vi "emi_Get system Info.vi"(11 "error in (no error)":errorcluster) -> (4 "Info retreived":bool, 8 "System Info":string, 15 "error out":errorcluster)   [LabVIEW 2011]
doc: "Reads a system infor summery from the OS.\n\nFor use in diagnostic files and such. \n\nThe system info generation takes a long time, so it should be run one time during startup. When it has run once, it will use the information retreived for all subsequent runs. First run: Long time. Secound run: No time.\nThe VI disregards the error input, and output. The asumption is that if this fails, the correct action is to do nothing. (The software should not exit due to this)."
uses:
  <vilib>/Utility/sysdir.llb/System Directory Type.ctl
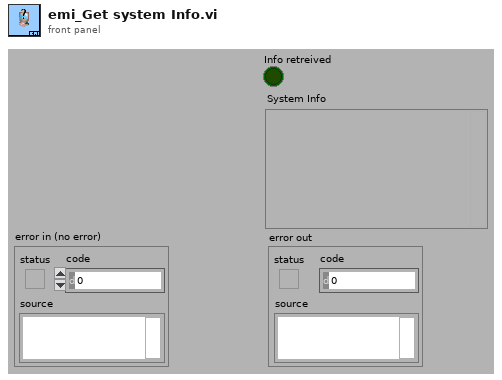
[diagram p1: front panel]
types:
  T1 = enum16{"open", "replace", "create", "open or create", "replace or create", "replace or create with confirmation"}
  T2 = typedef "System Directory Type.ctl" = i32
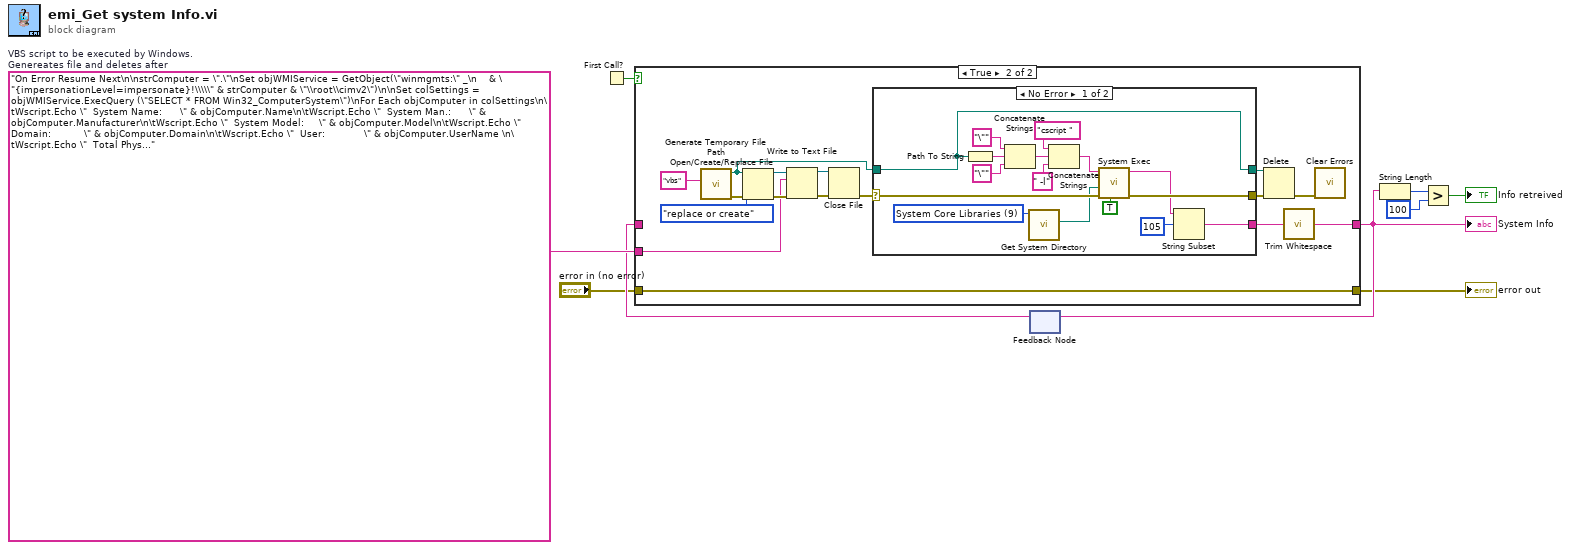
[diagram p0: block diagram]
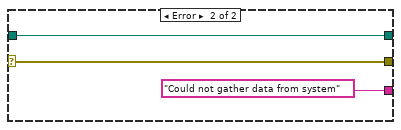
[diagram p3: hidden frame]
diagram:
  w9 = "On Error Resume Next\n\nstrComputer = \".\"\nSet objWMIService = GetObject(\"winmgmts:\" _\n    & \"{impersonationLevel=impersonate}!\\\\\" & strComputer & \"\\root\\cimv2\")\n\nSet colSettings = objWMIService.ExecQuery (\"SELECT * FROM Win32_ComputerSystem\")\nFor Each objComputer in colSettings\n\tWscript.Echo \"  System Name:      \" & objComputer.Name\n\tWscript.Echo \"  System Man.:      \" & objComputer.Manufacturer\n\tWscript.Echo \"  System Model:     \" & objComputer.Model\n\tWscript.Echo \"  Domain:           \" & objComputer.Domain\n\tWscript.Echo \"  User:             \" & objComputer.UserName \n\tWscript.Echo \"  Total Phys. Mem:  \" & objComputer.TotalPhysicalMemory\nNext\n\nSet colItems = objWMIService.ExecQuery(\"SELECT * FROM Win32_OperatingSystem\")\nFor Each objOperatingSystem in colItems \n \tWscript.Echo \"  Avail. Phys. Mem: \" & objOperatingSystem.FreePhysicalMemory\n \tWscript.Echo \"  Total Virt. Mem:  \" & objOperatingSystem.TotalVirtualMemorySize\n\tWscript.Echo \"  Avail. Virt. Mem: \" & objOperatingSystem.FreeVirtualMemory\n\tWscript.Echo \"  OS Name:          \" & objOperatingSystem.Name\n\tWscript.Echo \"  Version:          \" & objOperatingSystem.Version & \" SP: \" & objOperatingSystem.ServicePackMajorVersion & \".\" & objOperatingSystem.ServicePackMinorVersion\nNext\n\n\tWscript.Echo \" \"\n\nSet colItems = objWMIService.ExecQuery(\"Select * from Win32_SystemEnclosure\")\nFor Each objItem in colItems\n\tWscript.Echo \"  Part Numb.:       \" & objItem.PartNumber\n\tWscript.Echo \"  Serial Numb.:     \" & objItem.SerialNumber\n\tWscript.Echo \"  Asset tag.:       \" & objItem.SMBIOSAssetTag\nNext\n\n\tWscript.Echo \" \"\n\nSet colSettings = objWMIService.ExecQuery (\"SELECT * FROM Win32_ComputerSystem\")\nFor Each objComputer in colSettings\n\tWscript.Echo \"  Numb. CPU(s):     \" & objComputer.NumberOfProcessors\nNext\nSet colItems = objWMIService.ExecQuery(\"Select * from Win32_Processor\")\nFor Each objItem in colItems\n\tWscript.Echo \"  CPU Name:         \" & objItem.Name\n\tWscript.Echo \"    CPU Desc:       \" & objItem.Description\n\tWscript.Echo \"    L2 Cache:       \" & objItem.L2CacheSize & \" \" & objItem.L2CacheSpeed\n\tWscript.Echo \"    Clock speed:    \" & objItem.CurrentClockSpeed & \" (\" & objItem.MaxClockSpeed & \")\"\n\tWscript.Echo \"    Ext. Clock:     \" & objItem.ExtClock\n\tWscript.Echo \"    CPU Cores:      \" & objItem.NumberOfCores\n\tWscript.Echo \"    Logical CPUs:   \" & objItem.NumberOfLogicalProcessors\n\tWscript.Echo \"    CPU Version:   \" & objItem.Version & \" Rev: \" & objItem.Revision\nNext\n\n\tWscript.Echo \" \"\n\nSet colItems = objWMIService.ExecQuery(\"Select * from Win32_NetworkAdapterConfiguration\")\nFor Each objItem in colItems\n    If Not IsNull(objItem.IPAddress) Then \n        For i=LBound(objItem.IPAddress) to UBound(objItem.IPAddress)\n\t                Wscript.Echo \"  Adapter:          \" & objItem.Description \n\t                Wscript.Echo \"    Mac Addr.:      \" & objItem.MACAddress \n\t                Wscript.Echo \"    IP Address:     \" & objItem.IPAddress(i) \n\t                Wscript.Echo \"    IP Gateway:     \" & objItem.DefaultIPGateway(i)\n\t                Wscript.Echo \"    IP Subnet:      \" & objItem.IPSubnet(i) \n        Next\n    End If\nNext\n\n\tWscript.Echo \" \"\n\nComputerName = \".\"\nSet wmiServices  = GetObject ( _\n    \"winmgmts:{impersonationLevel=Impersonate}!//\" _\n    & ComputerName)\n' Get physical disk drive\nSet wmiDiskDrives =  wmiServices.ExecQuery ( _\n    \"SELECT Caption, DeviceID, SerialNumber FROM Win32_DiskDrive\")\n\nFor Each wmiDiskDrive In wmiDiskDrives\n    WScript.Echo \"  Drive: \" & wmiDiskDrive.Caption \n    WScript.Echo  \"    DeviceID: \" & \" (\" & wmiDiskDrive.DeviceID & \")\"\n    WScript.Echo  \"    Serial no: \" & wmiDiskDrive.SerialNumber\n    WScript.Echo \"    \" & wmiDiskPartition.DeviceID\n    'Use the disk drive device id to\n    ' find associated partition\n    query = \"ASSOCIATORS OF {Win32_DiskDrive.DeviceID='\" _\n        & wmiDiskDrive.DeviceID & \"'} WHERE AssocClass = Win32_DiskDriveToDiskPartition\"    \n    Set wmiDiskPartitions = wmiServices.ExecQuery(query)\n\n    For Each wmiDiskPartition In wmiDiskPartitions\n        'Use partition device id to find logical disk\n        Set wmiLogicalDisks = wmiServices.ExecQuery _\n            (\"ASSOCIATORS OF {Win32_DiskPartition.DeviceID='\" _\n             & wmiDiskPartition.DeviceID & \"'} WHERE AssocClass = Win32_LogicalDiskToPartition\") \n\n        For Each wmiLogicalDisk In wmiLogicalDisks\n            WScript.Echo \"    \" & wmiLogicalDisk.DeviceID & \"              \" &   wmiDiskPartition.DeviceID & \"    \" & _\n              wmiLogicalDisk.VolumeSerialNumber & \"    \" &  wmiLogicalDisk.FileSystem & \"    \" & wmiLogicalDisk.VolumeName\n        Next      \n    Next\nNext\n\n\tWscript.Echo \" \"\n\nSet colItems = objWMIService.ExecQuery(\"Select * from Win32_PnPSignedDriver\")\n\nFor Each objItem in colItems\nIf objItem.ClassGuid = \"{4d36e978-e325-11ce-bfc1-08002be10318}\" Then\n    Wscript.Echo \"  Port Name:         \" & objItem.FriendlyName\n    Wscript.Echo \"    Manufacturer:    \" & objItem.Manufacturer \n    Wscript.Echo \"    Device ID:       \" & objItem.DeviceID\n    Wscript.Echo \"    Driver Provider: \" & objItem.DriverProviderName\n    Wscript.Echo \"    Driver Version:  \" & objItem.DriverVersion\n    Wscript.Echo \"    INF Name:        \" & objItem.InfName\n    Wscript.Echo \"    Is Signed:       \" & objItem.IsSigned\n   End If \nNext\n\n\n\n\tWscript.Echo \" \"\n\tWscript.Echo \"SYSTEM ITEMS WITH ISSUES:\"\n\tWscript.Echo \" \"\n\nSet colItems = objWMIService.ExecQuery(\"Select * from Win32_PnPEntity WHERE ConfigManagerErrorCode <> 0\")\nFor Each objItem in colItems\n    Wscript.Echo \"  Description:      \" & objItem.Description\n    Wscript.Echo \"    Error Code:     \" & objItem.ConfigManagerErrorCode\n    Wscript.Echo \"    Class GUID:     \" & objItem.ClassGuid\n    Wscript.Echo \"    Device ID:      \" & objItem.DeviceID\n    Wscript.Echo \"    Manufacturer:   \" & objItem.Manufacturer\n    Wscript.Echo \"    Name:           \" & objItem.Name\n    Wscript.Echo \"    PNP Device ID:  \" & objItem.PNPDeviceID\n    Wscript.Echo \"    Service:        \" & objItem.Service\n\nNext\n\n\n\n"  # VBS script to be executed by Windows. Genereates file and deletes after
  n1 = First Call?() -> (First Call?: T/F=w8:bool)
  n2 = feedback #1() -> (w7:string)  [unwired: 1 in]
  n3 = case shown="True" w8 {
    tunnel: w9 -> [_ w23]
    tunnel: [w11 w13] -> w6
    tunnel: w7 -> [w11 _]
    tunnel: [w10 w12] -> w2
    tunnel: "error in (no error)" -> [w10 w12]
    frame False {
    }
    frame True {
      n4 = call <vilib>:"Generate Temporary File Path.vi"("Temporary File Extension (tmp)"="vbs") -> ("error out"=w26:errorcluster, "Unique Temporary File Path"=w16:path)  [unwired: 9 in]
      n5 = Open/Create/Replace File(file path (use dialog)=w16, error in=w26, operation (0:open)=T1."replace or create") -> (refnum out=w24:refnum<file>, error out=w25:errorcluster)  [unwired: 3 in, 1 out]
      n6 = Write to Text File(file (use dialog)=w24, text=w23, error in=w25) -> (refnum out=w21:refnum<file>, error out=w22:errorcluster)  [unwired: 1 in, 1 out]
      n7 = Close File(refnum=w21, error in=w22) -> (error out=w20:errorcluster)  [unwired: 1 out]
      n8 = case shown="No Error" w20 {
        selector: w20 -> [w30 w46]
        tunnel: w16 -> [w34 w45]
        tunnel: [w35 w46] -> w18
        tunnel: [w34 w45] -> w19
        tunnel: [w31 "Could not gather data from system" ("standard output")] -> w14
        frame No Error {
          w29 = T2 9 items=["User Home", "User Desktop", "User Documents", "User Application Data", "User Preferences", "User Temporary", "Public Documents", "Public Application Data", "Public Preferences", "System Core Libraries", "System Installed Libraries", "Application Files", "Boot Volume Root"] ("system directory type")
          n9 = Path To String(path=w34) -> (string=w36:string)
          n10 = Concatenate Strings("\"" ("string"), w36, "\"" ("string")) -> (w40:string)
          n11 = call <vilib>:"Get System Directory.vi"("system directory type"=w29) -> ("system directory"=w28:path)  [unwired: 10 in]
          n12 = Concatenate Strings("cscript " ("string"), w40, " -l" ("string")) -> (w37:string)
          n13 = call <vilib>:"System Exec.vi"("run minimized? (F)"=TRUE, "error in (no error)"=w30, "working directory"=w28, "command line"=w37) -> ("error out"=w35:errorcluster, "standard output"=w32:string)  [unwired: 2 in, 4 out]
          n14 = String Subset(string=w32, offset (0)=105 ("length (rest)")) -> (substring=w31:string)  [unwired: 1 in]
        }
        frame Error {
        }
      }
      n15 = Delete(path (use dialog)=w19, error in=w18) -> (error out=w17:errorcluster)  [unwired: 3 in, 2 out]
      n16 = call <vilib>:"Trim Whitespace.vi"("string"=w14) -> ("trimmed string"=w13:string)  [unwired: 1 in]
      n17 = call <vilib>:"Clear Errors.vi"("error in (no error)"=w17) -> ()  [unwired: 6 in, 1 out]
    }
  }
  "System Info" <- w6
  "error out" <- w2
  n18 = feedback-in #1(w6) -> ()
  n19 = String Length(string=w6) -> (length=w5:i32)
  n20 = Greater?(x=w5, y=100) -> (0:→"Info retreived":bool)
